vi "Global - All Loop Stop.vi"() -> ()   [LabVIEW 2014]
panel:
  in  "All Loop Stop":bool
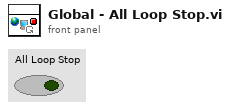
[diagram p1: front panel]
diagram:
